vi "Configure Trigger.vi"(8 "error in (no error)":errorcluster, 9 "Trigger Delay Mode (1: ON)":i32(ring)=1 items=["OFF", "ON", "ONCE"], 10 "Trigger Source (2: Immediate)":i32(ring)=2 items=["BUS", "HOLD", "IMM"], 11 "VISA resource name":refnum<visa-resource-name>) -> (0 "error out":errorcluster, 3 "VISA resource name out":refnum<visa-resource-name>)   [LabVIEW 2011, in "Agilent N432A.lvlib"]
doc: "Controls the behavior of Trigger Source and Trigger Delay."
uses:
  <instrlib>/Agilent N432A/Agilent N432A.lvlib
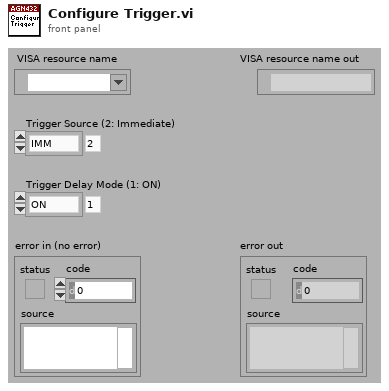
[diagram p1: front panel]
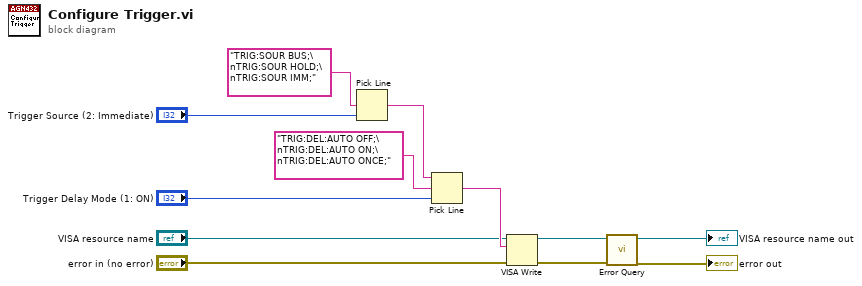
[diagram p0: block diagram]
diagram:
  n1 = Pick Line(multi-line string="TRIG:SOUR BUS;\nTRIG:SOUR HOLD;\nTRIG:SOUR IMM;", line index="Trigger Source (2: Immediate)") -> (output string=w8:string)  [unwired: 1 in]
  n2 = Pick Line(string ("")=w8, multi-line string="TRIG:DEL:AUTO OFF;\nTRIG:DEL:AUTO ON;\nTRIG:DEL:AUTO ONCE;", line index="Trigger Delay Mode (1: ON)") -> (output string=w7:string)
  n3 = VISA Write(VISA resource name="VISA resource name", write buffer=w7, error in (no error)="error in (no error)") -> (VISA resource name out=w4:refnum<visa-resource-name>, error out=w3:errorcluster)  [unwired: 1 out]
  n4 = call <instrlib>:"Error Query.vi"("error in (no error)"=w3, "VISA resource name"=w4) -> ("error out"=→"error out":errorcluster, "VISA resource name out"=→"VISA resource name out":refnum<visa-resource-name>)  [unwired: 6 in, 2 out]
